vi "Read.vi"(8 "error in (no error)":errorcluster) -> (0 "Data Frame":u8[](array[numeric]), 1 "Status":u8, 2 "error out":errorcluster)   [LabVIEW 2016]
uses:
  FPGA Bitfiles/FPGA_defref.ctl
panel:
  in  "FPGA VI Reference In":T1
  out "FPGA VI Reference Out":T1
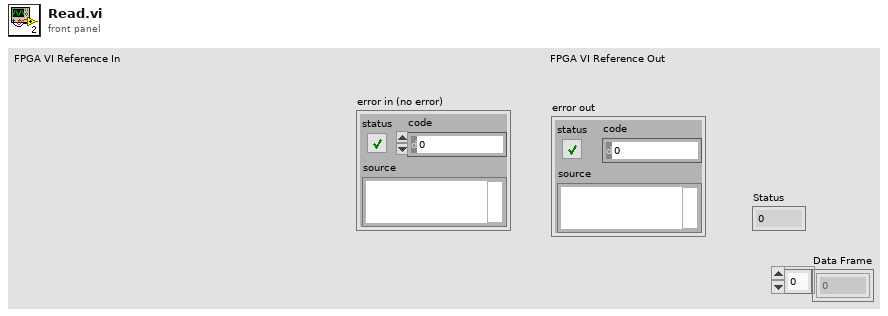
[diagram p1: front panel]
types:
  T1 = typedef "FPGA_defref.ctl" = refnum<k20>
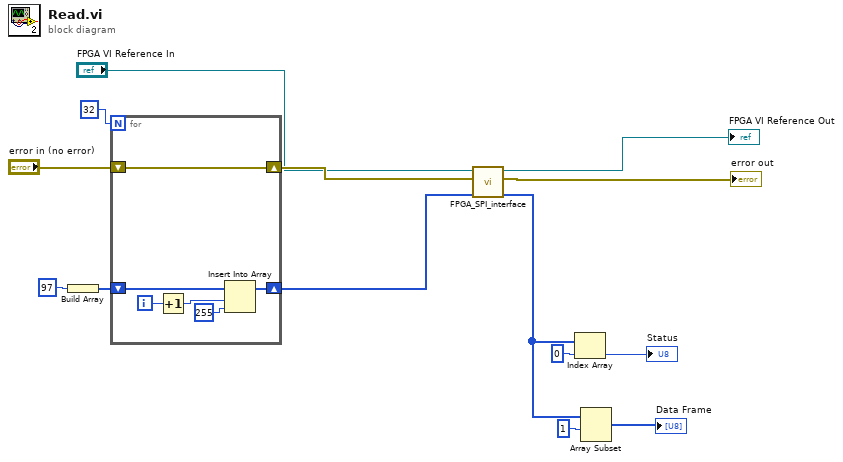
[diagram p0: block diagram]
diagram:
  n1 = Build Array(97) -> (w13:i32[])
  n2 = for {
    N: 32 -> [_]
    shift-right: [w18] -> w4
    shift-left: w13 -> [w19]
    shift-right: [w15] -> w6
    shift-left: "error in (no error)" -> [w15]
    i -> [w17]
    n3 = Increment(x=w17) -> (x+1=w16:i32)
    n4 = Insert Into Array(array=w19, index=w16, new element=255) -> (w18:i32[])
  }
  n5 = call "FPGA_SPI_interface.vi"("Frames to Write"=w4, "error in"=w6, "FPGA VI Reference In"="FPGA VI Reference In") -> ("Frames Read"=w3:u8[], "error out"=→"error out":errorcluster, "FPGA VI Reference Out"=→"FPGA VI Reference Out":T1)  [unwired: 6 in]
  n6 = Index Array(array=w3, index=0) -> (element=→"Status":u8)
  n7 = Array Subset(array=w3, index=1) -> (→"Data Frame":u8[])  [unwired: 1 in]
